vi "CONF Create digital tasks.vi"(7 "Config Digital Channels":T2={"SEnable"="line2", "SData"="line0", "SClock"="line1"}, 8 "error in (no error)":errorcluster, 10 "device in":tag="Dev1") -> (0 "error out":errorcluster, 3 "Digital ref out":T1)   [LabVIEW 2013]
uses:
  Kontrolki/KartaDAQ/CONF digital channel config.ctl
  Kontrolki/KartaDAQ/CONF Digital Refnum.ctl
  <vilib>/DAQmx/create/channels.llb/DAQmx Create Channel (DO-Digital Output).vi
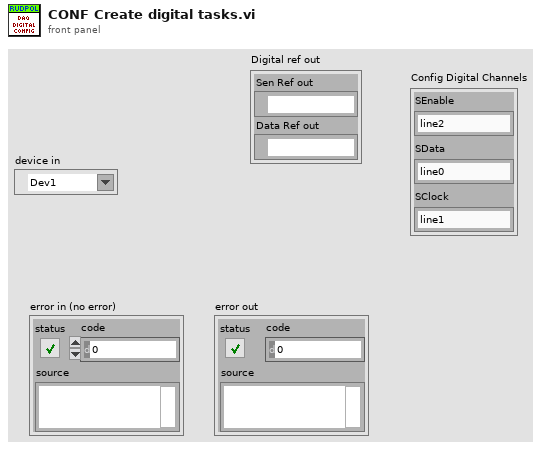
[diagram p1: front panel]
types:
  T1 = typedef "CONF Digital Refnum.ctl" = cluster{"Sen Ref out":refnum<k21>, "Data Ref out":refnum<k21>}
  T2 = typedef "CONF digital channel config.ctl" = cluster{"SEnable":string, "SData":string, "SClock":string}
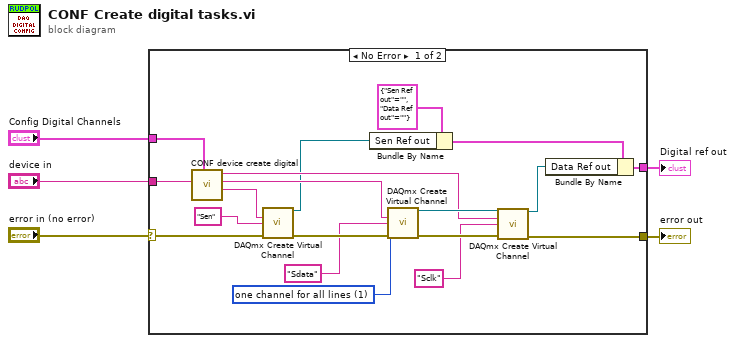
[diagram p0: block diagram]
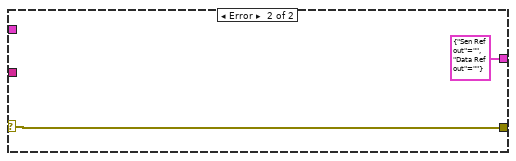
[diagram p2: hidden frame]
diagram:
  n1 = case shown="No Error" "error in (no error)" {
    selector: "error in (no error)" -> [w6 w26]
    tunnel: [w24 w26] -> w5
    tunnel: "Config Digital Channels" -> [w16 _]
    tunnel: "device in" -> [w15 _]
    tunnel: [w7 T1 {"Sen Ref out"="", "Data Ref out"=""} ("Digital ref out")] -> w2
    frame No Error {
      w20 = 1 items=["one channel for each line", "one channel for all lines"] ("line grouping")
      n2 = call "CONF device create digital.vi"("Config Digital Channels"=w16, "device in"=w15) -> ("Sen"=w14:tag, "Sdata"=w13:tag, "Scl"=w12:tag)  [unwired: 7 in]
      n3 = call-poly <vilib>:"DAQmx Create Virtual Channel.vi"("lines"=w14, "name to assign"="Sen", "error in"=w6) -> ("task out"=w10:refnum<k21>, "error out"=w23:errorcluster)  [unwired: 11 in]
      n4 = Bundle By Name(cluster=T1 {"Sen Ref out"="", "Data Ref out"=""} ("Digital ref out"), "Sen Ref out"=w10) -> (w9:T1)
      n5 = call-poly <vilib>:"DAQmx Create Virtual Channel.vi"("lines"=w13, "name to assign"="Sdata", "line grouping"=w20, "error in"=w23) -> ("task out"=w18:refnum<k21>, "error out"=w19:errorcluster)  [unwired: 10 in]
      n6 = call-poly <vilib>:"DAQmx Create Virtual Channel.vi"("task in"=w18, "lines"=w12, "name to assign"="Sclk", "error in"=w19) -> ("task out"=w8:refnum<k21>, "error out"=w24:errorcluster)  [unwired: 10 in]
      n7 = Bundle By Name(cluster=w9, "Data Ref out"=w8) -> (w7:T1)
    }
    frame Error {
    }
  }
  "error out" <- w5
  "Digital ref out" <- w2
